vi "OE2031&OE2041_USB_Query Data.vi"(0 "VISA resource name":refnum<visa-resource-name>, 11 "Error in (no error)":errorcluster caption="error out（no error）") -> (3 "Buffer Count":u8, 4 "VISA resource  out":refnum<visa-resource-name>, 6 "Total Data Array":dbl[][](array[numeric]), 8 "Parameter Values":T2, 10 "Output String":string, 13 "PLL&Overload":T1, 14 "Trig In_Count":u8[](array[numeric]), 15 "Error out":errorcluster caption="error out")   [LabVIEW 2011]
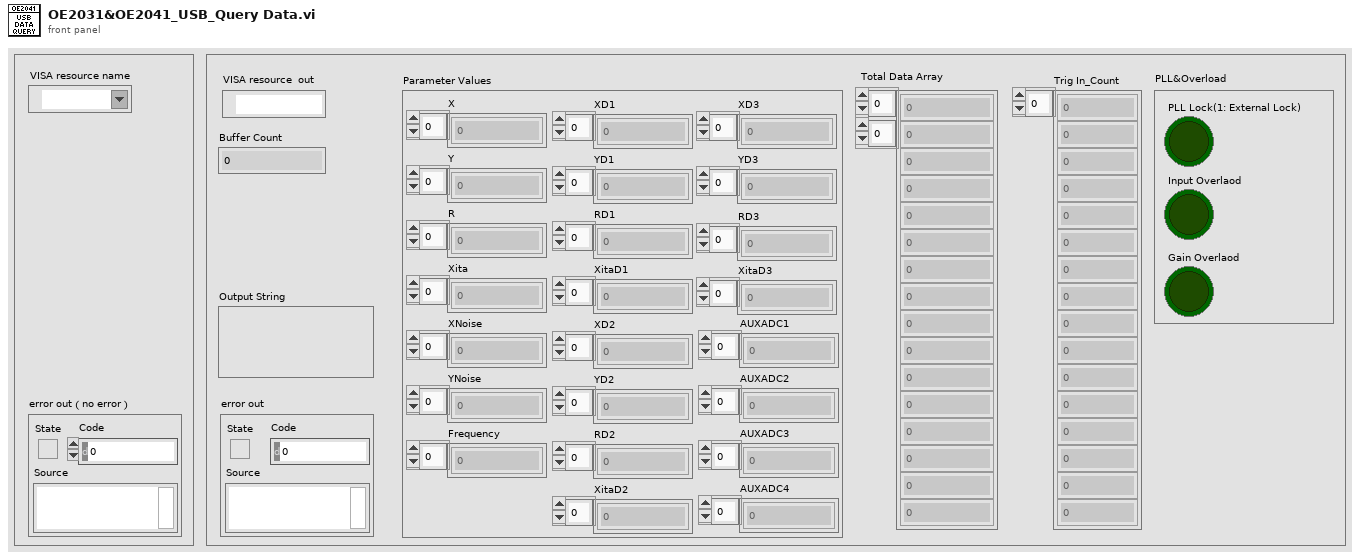
[diagram p1: front panel]
types:
  T1 = cluster{"PLL Lock(1: External Lock)":bool, "Input Overlaod":bool, "Gain Overlaod":bool}
  T2 = cluster{"X":dbl[], "Y":dbl[], "R":dbl[], "Xita":dbl[], "XNoise":dbl[], "YNoise":dbl[], "Frequency":dbl[], "XD1":dbl[], "YD1":dbl[], "RD1":dbl[], "XitaD1":dbl[], "XD2":dbl[], "YD2":dbl[], "RD2":dbl[], "XitaD2":dbl[], "XD3":dbl[], "YD3":dbl[], "RD3":dbl[], "XitaD3":dbl[], "AUXADC1":dbl[], "AUXADC2":dbl[], "AUXADC3":dbl[], "AUXADC4":dbl[]}
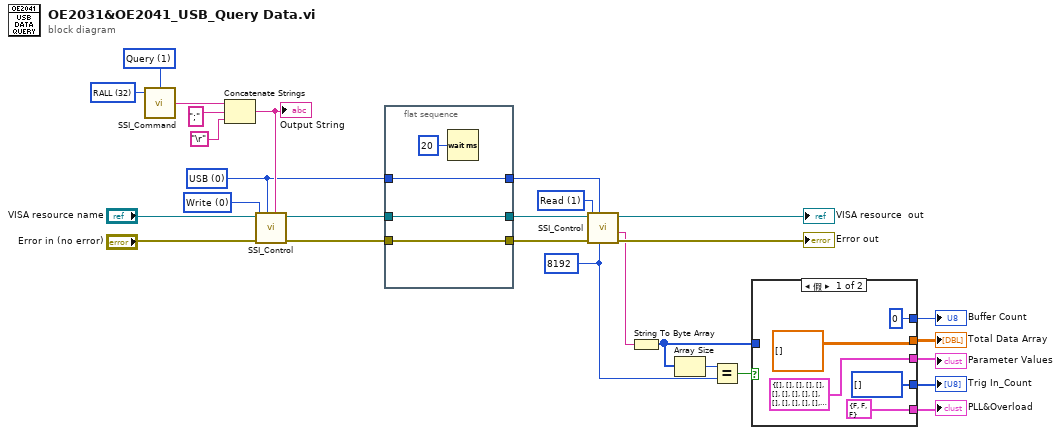
[diagram p0: block diagram]
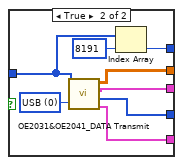
[diagram p2: hidden frame]
diagram:
  w14 = u32 8192 ("Number of bytes")
  w17 = u16 1 items=["Write", "Read"] ("Control")
  w6 = u16 0 items=["USB", "RS232", "GPIB", "Ethernet"] ("Remote Mode")
  w19 = u16 0 items=["Write", "Read"] ("Control")
  w24 = u16 32 items=["ISRC", "IGND", "ICPL", "ILIN", "PHAS", "FMOD", "RSLP", "FREQ", "SWPT", "SLLM", "SULM", "SSLL", "SSLG", "STLM", "SWRM", "IRNG", "SENS", "RMOD", "OFLT", "OFSL", "SYNC", "DMOD", "HARM", "DARB", "SWVT", "SLVL", "SVLL", "SVUL", "SVSL", "SVSG", "SVTM", "SVRM", "RALL", "SNAP", "OUTP", "OAUX", "COUT", "CAUX", "COFP", "CEXP", "FPOP", "OEXP", "*IDN", "*RST", "OVLD", "INOV", "GNOV", "*PLL", "SSET", "RSET", "AGAN", "APHS", "ARSV", "ASCL", "EQCD", "EQCS", "SPED", "SRAT", "SLEN", "SSLE", "STRG", "SPRM", "STRD", "PAUS", "RSET", "SPTS", "TRCA", "TEMP", "RSTU", "INHZ", "DEQU", "SADD", "ARNG", "CSPE", "ISRCD", "IGNDD", "ICPLD", "ILIND", "PHASD", "FMODD", "RSLPD", "FREQD", "SWPTD", "SLLMD", "SULMD", "SSLLD", "SSLGD", "STLMD", "SWRMD", "SENSD", "RMODD", "OFLTD", "OFSLD", "SYNCD", "HARMD", "EQCDD", "EQCSD", "SNAPD", "OUTPD", "SWVTD", "SLVLD", "SVLLD", "SVULD", "SVSLD", "SVSGD", "SVTMD", "SVRMD", "SVDCD", "ARSVD", "AGAND", "APHSD", "ASCLD", "FPOPD", "CAUXD", "OEXPD", "SPEDD", "SRATD", "SLEND", "SSLED", "STRGD", "SPRMD", "STRDD", "PAUSD", "RESTD", "SPTSD", "TRCAD", "*IDND", "*RSTD", "INOVD", "GNOVD", "*PLLD", "SSETD", "RSETD", "RALLD"] ("Command Type")
  w22 = u16 1 items=["Set", "Query"] ("Opera")
  n1 = call "SSI_Command.vi"("Opera"=w22, "Command Type"=w24) -> ("Output string"=w25:string)  [unwired: 2 in]
  n2 = Concatenate Strings(w25, ";" ("字符串"), "\r") -> (w28:string)
  "Output String" <- w28
  n3 = call "SSI_Control.vi"("Write Buffer"=w28, "Remote Mode"=w6, "Error in (no error)"="Error in (no error)", "Control"=w19, "VISA resource name"="VISA resource name") -> ("Error out"=w3:errorcluster, "VISA resource  out"=w4:refnum<visa-resource-name>)  [unwired: 3 in, 2 out]
  n4 = flat-sequence {
    tunnel: [w31] -> w5
    tunnel: w6 -> [w31]
    tunnel: [w30] -> w1
    tunnel: w4 -> [w30]
    tunnel: [w29] -> w2
    tunnel: w3 -> [w29]
    frame #0 {
      n5 = Wait (ms)(milliseconds to wait=u32 20 ("等待时间（毫秒）")) -> ()  [unwired: 1 out]
    }
  }
  n6 = call "SSI_Control.vi"("Number of bytes"=w14, "Remote Mode"=w5, "Error in (no error)"=w2, "Control"=w17, "VISA resource name"=w1) -> ("Error out"=→"Error out":errorcluster, "Read Buffer"=w15:string, "VISA resource  out"=→"VISA resource  out":refnum<visa-resource-name>)  [unwired: 3 in, 1 out]
  n7 = String To Byte Array(string=w15) -> (unsigned byte array=w8:u8[])
  n8 = Array Size(array=w8) -> (size(s)=w9:i32)
  n9 = Equal?(x=w9, y=w14) -> (x = y?=w10:bool)
  n10 = case shown="假" w10 {
    tunnel: [T2 {"X"=[], "Y"=[], "R"=[], "Xita"=[], "XNoise"=[], "YNoise"=[], "Frequency"=[], "XD1"=[], "YD1"=[], "RD1"=[], "XitaD1"=[], "XD2"=[], "YD2"=[], "RD2"=[], "XitaD2"=[], "XD3"=[], "YD3"=[], "RD3"=[], "XitaD3"=[], "AUXADC1"=[], "AUXADC2"=[], "AUXADC3"=[], "AUXADC4"=[]} ("Parameter Values") w40] -> w13
    tunnel: [dbl[][] [] ("Total Data Array") w41] -> w27
    tunnel: [u8 0 w44] -> w12
    tunnel: [u8[] [] ("Trig_Count") w39] -> w11
    tunnel: w8 -> [_ w42]
    tunnel: [T1 {"PLL Lock(1: External Lock)"=FALSE, "Input Overlaod"=FALSE, "Gain Overlaod"=FALSE} ("PLL&Overload") w38] -> w7
    frame False {
    }
    frame True {
      w43 = u16 0 items=["USB"=0, "Ethernet"=3] ("Remote Mode")
      n11 = call "OE2031&OE2041_DATA Transmit.vi"("Input Data"=w42, "Remote Mode"=w43) -> ("Total Data Array"=w41:dbl[][], "Parameter Values"=w40:T2, "Trig_Count"=w39:u8[], "PLL&Overload"=w38:T1)
      n12 = Index Array(array=w42, index=8191 ("索引")) -> (element=w44:u8)
    }
  }
  "Parameter Values" <- w13
  "Total Data Array" <- w27
  "Buffer Count" <- w12
  "Trig In_Count" <- w11
  "PLL&Overload" <- w7
